vi "Trim Whitespace.vi"(3 "String in":string) -> (1 "Trimmed":string)   [LabVIEW 2020, in "CTI.lvlib"]
uses:
  CTI.lvlib
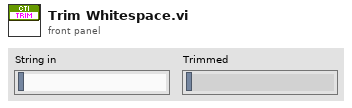
[diagram p1: front panel]
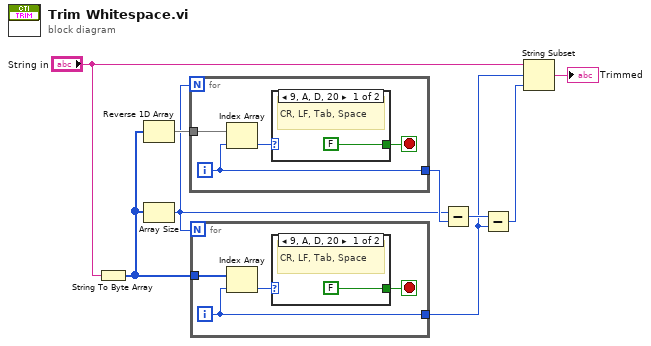
[diagram p0: block diagram]
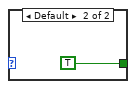
[diagram p2: hidden frame]
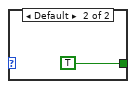
[diagram p3: hidden frame]
diagram:
  n1 = String To Byte Array(string="String in") -> (unsigned byte array=w8:u8[])
  n2 = Reverse 1D Array(array=w8) -> (reversed array=w9:u8[])
  n3 = Array Size(array=w8) -> (size(s)=w1:i32)
  n4 = for {
    N: w1 -> [_]
    tunnel: w9 -> [w13]
    tunnel: [w11] -> w7
    i -> [w11]
    stop <- w10 stop-if-true
    n5 = Index Array(array=w13, index=w11) -> (element=w12:u8)
    n6 = case shown="9, A, D, 20" w12 {
      tunnel: [FALSE TRUE] -> w10
      frame 9, 10, 13, 32 {
        # "CR, LF, Tab, Space"
      }
      frame Default {
      }
    }
  }
  n7 = for {
    N: w1 -> [_]
    tunnel: w8 -> [w19]
    tunnel: [w17] -> w4
    i -> [w17]
    stop <- w16 stop-if-true
    n8 = Index Array(array=w19, index=w17) -> (element=w18:u8)
    n9 = case shown="9, A, D, 20" w18 {
      tunnel: [FALSE TRUE] -> w16
      frame 9, 10, 13, 32 {
        # "CR, LF, Tab, Space"
      }
      frame Default {
      }
    }
  }
  n10 = Subtract(x=w1, y=w7) -> (x-y=w6:i32)
  n11 = Subtract(x=w6, y=w4) -> (x-y=w3:i32)
  n12 = String Subset(string="String in", offset (0)=w4, length (rest)=w3) -> (substring=→"Trimmed":string)
